vi "get_number_of_frames.vi"(8 "error in (no error)":errorcluster, 11 "ImagingModeDL090130Frame in":refnum<class "ImagingModeDL090130Frame.lvclass">=refnum) -> (0 "error out":errorcluster, 2 "number of frames":i32, 3 "ImagingModeDL090130Frame out":refnum<class "ImagingModeDL090130Frame.lvclass">)   [LabVIEW 2010, in "ImagingModeDL090130Frame.lvclass"]
uses:
  ImagingModeDL090130Frame.lvclass
  ImagingModeDL090130Frame.lvclass/ImagingModeDL090130Frame.ctl
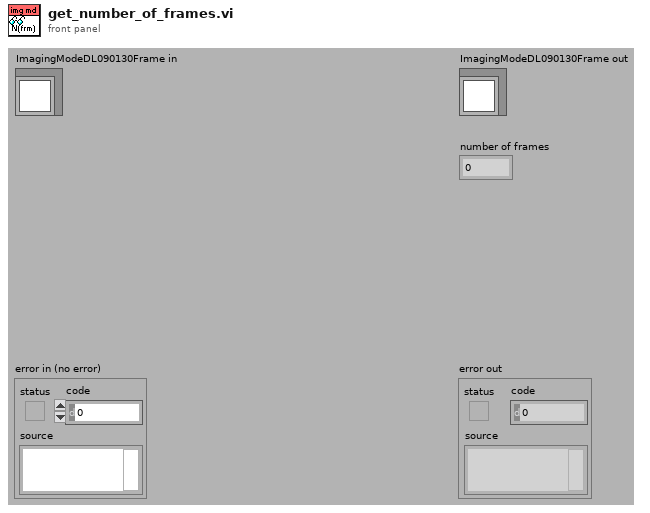
[diagram p1: front panel]
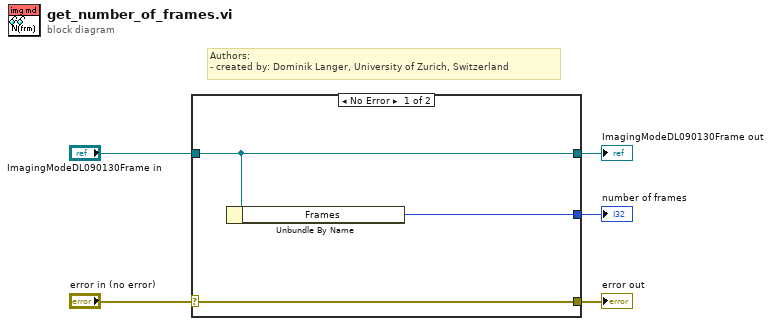
[diagram p0: block diagram]
diagram:
  # "Authors: \n- created by: Dominik Langer, University of Zurich, Switzerland"
  n1 = case shown="No Error" "error in (no error)" {
    selector: "error in (no error)" -> [w8 w9]
    tunnel: [w8 w9] -> w4
    tunnel: [w7 w10] -> w2
    tunnel: "ImagingModeDL090130Frame in" -> [w7 w10]
    tunnel: [w6 _] -> w1
    frame No Error {
      n2 = Unbundle By Name(w7) -> ("Frames"=w6:i32)
    }
    frame Error {
    }
  }
  "error out" <- w4
  "ImagingModeDL090130Frame out" <- w2
  "number of frames" <- w1
